vi "Actor Core.vi"(8 "error in":errorcluster, 11 "CS++DeviceGUIActor.lvclass":refnum<class "CS++DeviceGUIActor.lvclass">) -> (0 "error out":errorcluster, 3 "Actor out":refnum<class "Actor.lvclass">)   [LabVIEW 2013, in "CS++DeviceGUIActor.lvlib" / "CS++DeviceGUIActor.lvclass"]
doc: "(<B>Filename</B>: Actor Framework.lvlib:Actor.lvclass:Actor Core.vi)\n\nReceives messages to the actor, reacts to them, and initiates any error handling that may shut the actor down.\n\nDescendant classes may override this VI to append parallel tasks for the actor to complete while it handles messages. Overrides use the Call Parent Method node."
uses:
  CS++DeviceGUIActor.lvclass
  <vilib>/ActorFramework/Actor/Actor.lvclass
  CS++BaseActor/CS++BaseActor.lvclass/CS++BaseActor.ctl
  CS++DeviceGUIActor.lvclass/CS++DeviceGUIActor.ctl
  CS++GUIActor/CS++GUIActor.lvclass/CS++GUIActor.ctl
  Classes/CS++BaseClasses/Factory/CS++Factory.lvclass
  CS++GUIActor/CS++GUIActor.lvclass
  <vilib>/ActorFramework/Actor/Actor.lvclass/Actor.ctl
  <vilib>/ActorFramework/Message Enqueuer/Message Enqueuer.lvclass/Message Enqueuer.ctl
  <vilib>/ActorFramework/Message Enqueuer/Init from Existing Queue.vi
  <vilib>/ActorFramework/Message Enqueuer/Enqueue.vi
  <vilib>/ActorFramework/Message Priority Queue/Priority Enqueue.vi
  <vilib>/ActorFramework/Message Enqueuer/Message Enqueuer.lvclass
  <vilib>/ActorFramework/Stop Msg/Stop Msg.lvclass
  CS++BaseActor/CS++BaseActor.lvclass
panel:
  out "Resource Name":string
  out "Self-Test Result Message":string
  out "Self-Test Result Code":i32
  out "Firmware Revision":string
  out "Driver Revision":string
  in  "Stop Button":bool
  out "Actor Name":string
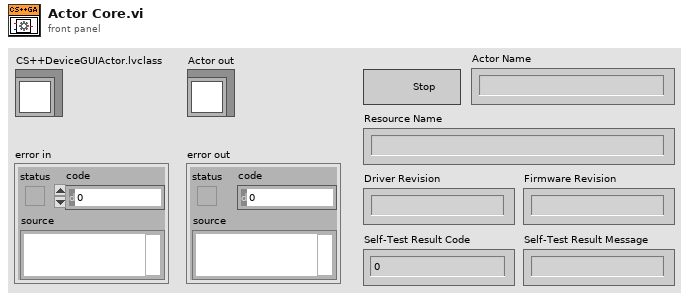
[diagram p1: front panel]
types:
  T1 = enum32{"Invalid", "Standard", "Closed", "Hidden", "Minimized", "Maximized"}
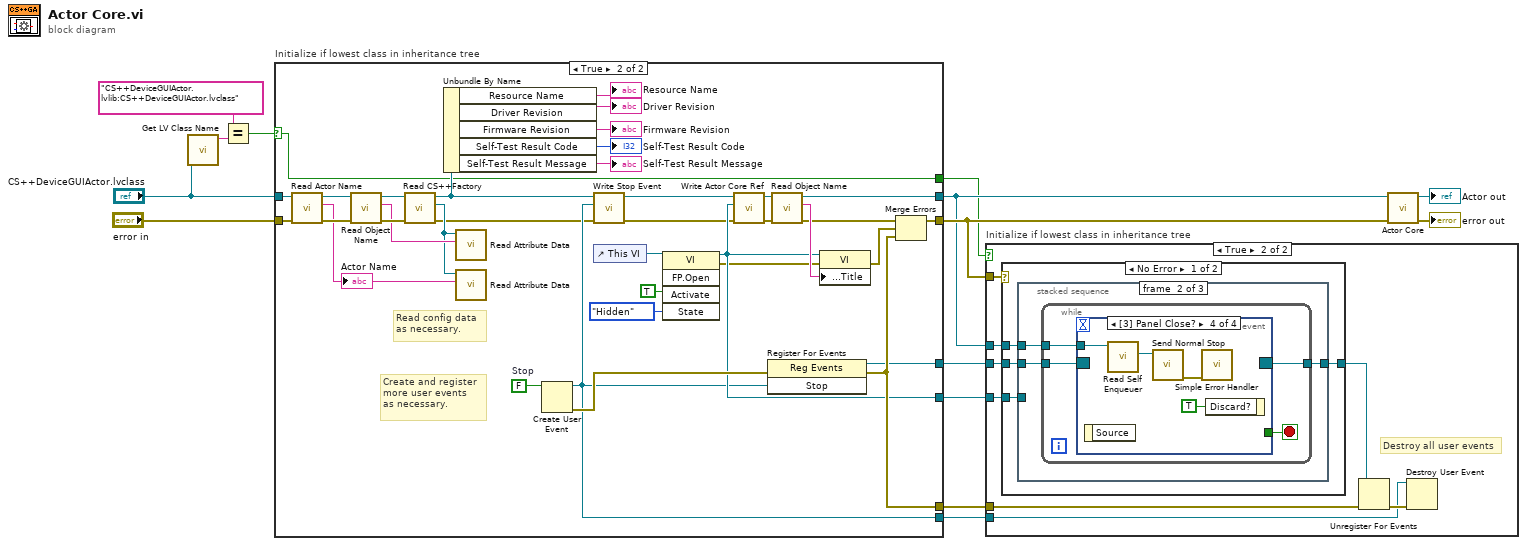
[diagram p0: block diagram]
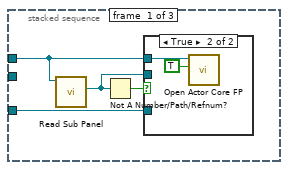
[diagram p4: hidden frame]
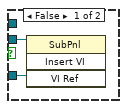
[diagram p5: hidden frame]
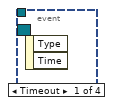
[diagram p6: hidden frame]
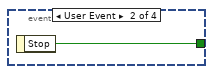
[diagram p7: hidden frame]
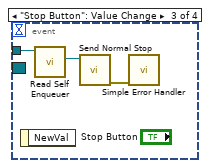
[diagram p8: hidden frame]
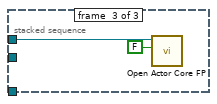
[diagram p9: hidden frame]
diagram:
  n1 = call <vilib>:"Get LV Class Name.vi"("object"="CS++DeviceGUIActor.lvclass") -> ("class name"=w8:string)  [unwired: 9 in, 1 out]
  n2 = Equal?(x="CS++DeviceGUIActor.lvlib:CS++DeviceGUIActor.lvclass" ("class name"), y=w8) -> (x = y?=w2:bool)
  n3 = case "Initialize if lowest class in inheritance tree" shown="True" w2 {
    selector: w2 -> [w15 w18]
    tunnel: [w16 w53] -> w12
    tunnel: "error in" -> [w16 w52]
    tunnel: [w17 w51] -> w10
    tunnel: "CS++DeviceGUIActor.lvclass" -> [w17 w50]
    tunnel: [_ w42] -> w6
    tunnel: [_ w41] -> w5
    tunnel: [_ w40] -> w4
    tunnel: [_ w31] -> w3
    tunnel: [w15 w18] -> w1
    frame False {
    }
    frame True {
      w45 = FALSE  # Stop
      # "Create and register \nmore user events\nas necessary."
      # "Read config data\nas necessary."
      n4 = call-dynamic "Read Actor Name.vi"("error in (no error)"=w52, "CS++GUIActor in"=w50) -> ("error out"=w34:errorcluster, "Actor Name"=w32:string, "CS++GUIActor out"=w35:refnum<class "CS++DeviceGUIActor.lvclass">)  [unwired: 7 in]
      "Actor Name" <- w32
      n5 = call "Read Object Name.vi"("error in (no error)"=w34, "CS++BaseActor in"=w35) -> ("error out"=w37:errorcluster, "Object Name"=w36:string, "CS++BaseActor out"=w38:refnum<class "CS++DeviceGUIActor.lvclass">)  [unwired: 7 in]
      n6 = call "Read CS++Factory.vi"("error in (no error)"=w37, "CS++BaseActor in"=w38) -> ("error out"=w30:errorcluster, "CS++Factory"=w33:refnum<class "CS++Factory.lvclass">, "CS++BaseActor out"=w24:refnum<class "CS++DeviceGUIActor.lvclass">)  [unwired: 7 in]
      n7 = Unbundle By Name(w24) -> ("Resource Name"=→"Resource Name":string, "Driver Revision"=→"Driver Revision":string, "Firmware Revision"=→"Firmware Revision":string, "Self-Test Result Code"=→"Self-Test Result Code":i32, "Self-Test Result Message"=→"Self-Test Result Message":string)
      n8 = call-dynamic "Read Attribute Data.vi"("Object Name"=w36, "CS++Factory in"=w33) -> ()  [unwired: 7 in, 3 out]
      n9 = call-dynamic "Read Attribute Data.vi"("Object Name"=w32, "CS++Factory in"=w33) -> ()  [unwired: 7 in, 3 out]
      n10 = Create User Event(user event datatype=w45) -> (user event=w31:refnum<user-event>, error out=w43:errorcluster)  [unwired: 1 in]
      n11 = call "Write Stop Event.vi"("error in (no error)"=w30, "Stop"=w31, "CS++GUIActor in"=w24) -> ("error out"=w28:errorcluster, "CS++GUIActor out"=w29:refnum<class "CS++DeviceGUIActor.lvclass">)  [unwired: 7 in]
      n12 = control-ref of="This VI"() -> (w49:refnum<vi>)
      n13 = invoke class="VI" method="FP.Open"(reference=w49, "Activate"=TRUE ("Activate?"), "State"=T1."Hidden") -> (reference out=w40:refnum<vi>, error out=w39:errorcluster)  [unwired: 2 in, 3 out]
      n14 = call "Write Actor Core Ref.vi"("error in (no error)"=w28, "Actor Core Ref"=w40, "CS++BaseActor in"=w29) -> ("error out"=w27:errorcluster, "CS++BaseActor out"=w26:refnum<class "CS++DeviceGUIActor.lvclass">)  [unwired: 7 in]
      n15 = register-events(error in=w43, w31) -> (reference out=w41:refnum<event-registration>, error out=w42:errorcluster)  [unwired: 1 in]
      n16 = call "Read Object Name.vi"("error in (no error)"=w27, "CS++BaseActor in"=w26) -> ("error out"=w25:errorcluster, "Object Name"=w46:string, "CS++BaseActor out"=w51:refnum<class "CS++DeviceGUIActor.lvclass">)  [unwired: 7 in]
      n17 = property class="VI"(reference=w40, error in=w39, "Front Panel.Title"=w46) -> (error out=w44:errorcluster)  [unwired: 1 out]
      n18 = Merge Errors(w25, w44, w42) -> (w53:errorcluster)
    }
  }
  n19 = case "Initialize if lowest class in inheritance tree" shown="True" w1 {
    tunnel: w12 -> [_ w61]
    tunnel: w10 -> [_ w60]
    tunnel: w6 -> [_ w58]
    tunnel: w5 -> [_ w57]
    tunnel: w4 -> [_ w55]
    tunnel: w3 -> [_ w54]
    frame False {
    }
    frame True {
      # "Destroy all user events"
      n20 = case shown="No Error" w61 {
        tunnel: w60 -> [w65 _]
        tunnel: w57 -> [w64 w91]
        tunnel: [w63 w91] -> w56
        tunnel: w55 -> [w62 _]
        frame No Error {
          n21 = stacked-sequence {
            tunnel: w65 -> [w67 w75 w90]
            tunnel: w64 -> [_ w76 _]
            tunnel: [_ w74 _] -> w63
            tunnel: w62 -> [w68 _ _]
            frame #0 {
              n22 = call-dynamic "Read Sub Panel.vi"("CS++GUIActor in"=w67) -> ("Sub Panel"=w66:refnum<vi>)  [unwired: 8 in, 2 out]
              n23 = Not A Number/Path/Refnum?(number/path/refnum=w66) -> (NaN/Path/Refnum?=w69:bool)
              n24 = case shown="True" w69 {
                tunnel: w67 -> [_ w73]
                tunnel: w66 -> [w71 _]
                tunnel: w68 -> [w70 _]
                frame False {
                  n25 = invoke class="SubPnl" method="Insert VI"(reference=w71, "VI Ref"=w70) -> ()  [unwired: 2 in, 4 out]
                }
                frame True {
                  n26 = call "Open Actor Core FP.vi"("Open FP (F)"=TRUE, "CS++BaseActor in"=w73) -> ()  [unwired: 8 in, 2 out]
                }
              }
            }
            frame #1 {
              n27 = while {
                tunnel: w76 -> [w80]
                tunnel: w75 -> [w79]
                tunnel: [w77] -> w74
                stop <- w78 stop-if-true
                n28 = event shown="[3] Panel Close?" {
                  selector: w80 -> [_ _ _ _]
                  dyn-events: [_ _ _ _] -> w77
                  timeout: _ -> [_ _ _ _]
                  tunnel: w79 -> [_ _ w84 w85]
                  tunnel: [_ w81 _ _] -> w78
                  event Timeout {
                    n29 = event-data() -> ()  [unwired: 1 in, 2 out]
                  }
                  event User Event {
                    n30 = event-data() -> ("Stop"=w81:bool)  [unwired: 1 in]
                  }
                  event "Stop Button": Value Change {
                    n31 = event-data() -> ()  [unwired: 1 in, 1 out]
                    n32 = call <vilib>:"Read Self Enqueuer.vi"("Actor"=w84) -> ("Self Enqueuer"=w83:refnum<class "Message Enqueuer.lvclass">)  [unwired: 10 in]
                    n33 = call <vilib>:"Send Normal Stop.vi"("Message Enqueuer"=w83) -> ("error out"=w82:errorcluster)  [unwired: 10 in]
                    n34 = call <vilib>:"Simple Error Handler.vi"("error in (no error)"=w82) -> ()  [unwired: 4 in, 5 out]
                  }
                  event Panel Close? {
                    n35 = event-data() -> ()  [unwired: 1 in, 1 out]
                    n36 = call <vilib>:"Read Self Enqueuer.vi"("Actor"=w85) -> ("Self Enqueuer"=w87:refnum<class "Message Enqueuer.lvclass">)  [unwired: 10 in]
                    n37 = call <vilib>:"Send Normal Stop.vi"("Message Enqueuer"=w87) -> ("error out"=w86:errorcluster)  [unwired: 10 in]
                    n38 = call <vilib>:"Simple Error Handler.vi"("error in (no error)"=w86) -> ()  [unwired: 4 in, 5 out]
                    n39 = event-data("Discard?"=TRUE) -> ()  [unwired: 1 in, 1 out]
                  }
                }
              }
            }
            frame #2 {
              n40 = call "Open Actor Core FP.vi"("Open FP (F)"=FALSE, "CS++BaseActor in"=w90) -> ()  [unwired: 8 in, 2 out]
            }
          }
        }
        frame Error {
        }
      }
      n41 = Unregister For Events(event registration refnum=w56, error in=w58) -> (error out=w59:errorcluster)
      n42 = Destroy User Event(user event=w54, error in=w59) -> ()  [unwired: 1 out]
    }
  }
  n43 = call-parent "Actor Core.vi"("error in"=w12, "CS++GUIActor in"=w10) -> ("error out"=→"error out":errorcluster, "Actor out"=→"Actor out":refnum<class "Actor.lvclass">)  [unwired: 8 in]
